vi "TestAbstractTransport_Error.vi"(8 "error in (no error)":errorcluster, 11 "TestCase in":refnum<class "TestTransport.lvclass">) -> (0 "error out":errorcluster, 3 "TestCase out":refnum<class "TestTransport.lvclass">)   [LabVIEW 2015, in "Transport.lvlib" / "TestTransport.lvclass"]
uses:
  TestTransport.lvclass
  IMediator/ITransport/ITransport.lvclass
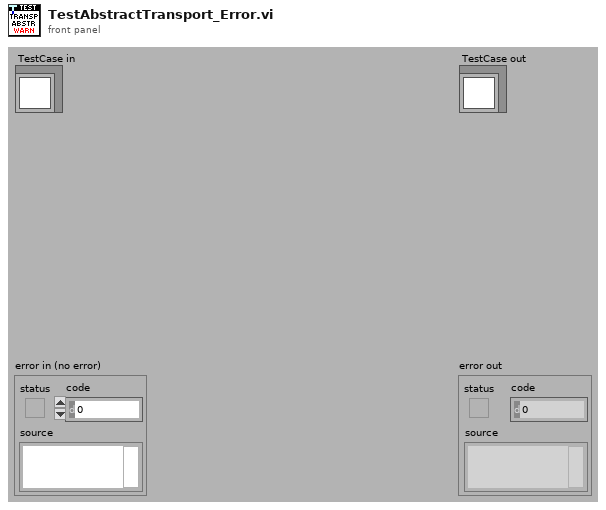
[diagram p1: front panel]
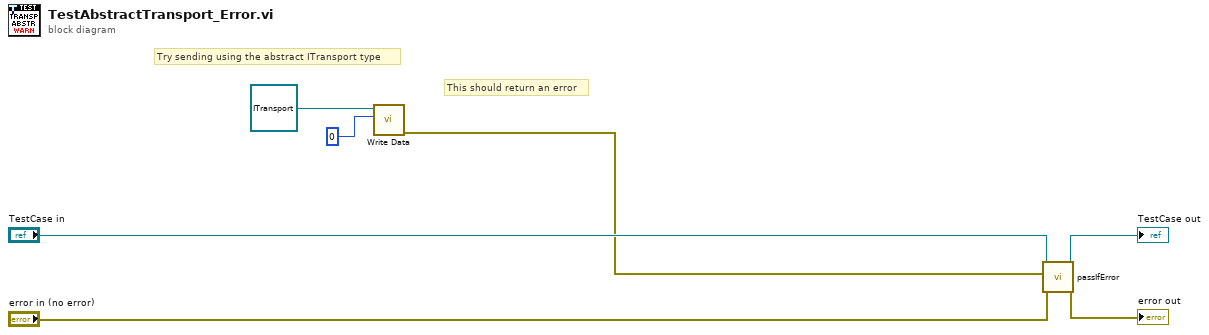
[diagram p0: block diagram]
diagram:
  # "This should return an error"
  # "Try sending using the abstract ITransport type"
  n1 = call-dynamic "Write Data.vi"("Value"=0, "ITransport in"=refnum<class "ITransport.lvclass"> refnum ("IMediator.lvlib:ITransport.lvclass")) -> ("error out"=w1:errorcluster)  [unwired: 8 in, 1 out]
  n2 = call-dynamic "passIfError.vi"("error in (no error)"="error in (no error)", "error"=w1, "TestCase in"="TestCase in") -> ("error out"=→"error out":errorcluster, "TestCase out"=→"TestCase out":refnum<class "TestTransport.lvclass">)  [unwired: 7 in]
